vi "2ComboKeyDetect (SubVI).vi"(9 "negKey":T1(ring), 10 "posKey":T1(ring), 11 "keys pressed":T2(array[ring])) -> (3 "speedout":dbl(slide) scale=-100.0..100.0)   [LabVIEW 2018]
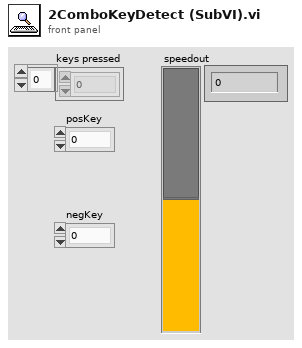
[diagram p1: front panel]
types:
  T1 = enum16{"0", "1", "2", "3", "4", "5", "6", "7", "8", "9", "A", "B", "C", "D", "E", "F", "G", "H", "I", "J", "K", "L", "M", "N", "O", "P", "Q", "R", "S", "T", "U", "V", "W", "X", "Y", "Z", "F1", "F2", "F3", "F4", "F5", "F6", "F7", "F8", "F9", "F10", "F11", "F12", "F13", "F14", "F15", "ADD", "BACK", "BACKSLASH", "CAPITAL", "COMMA", "DECIMAL", "DELETE", "DIVIDE", "DOWN", "END", "EQUALS", "ESCAPE", "GRAVE (`)", "HOME", "INSERT", "LBRACKET", "LCONTROL", "LEFT", "L ALT", "LSHIFT", "LWIN", "MINUS", "MULTIPLY", "NEXT", "NUMLOCK", "NUMPAD_0", "NUMPAD_1", "NUMPAD_2", "NUMPAD_3", "NUMPAD_4", "NUMPAD_5", "NUMPAD_6", "NUMPAD_7", "NUMPAD_8", "NUMPAD_9", "PAUSE", "PERIOD", "PRIOR (PG UP)", "RBRACKET", "RCONTROL", "RETURN", "RIGHT", "R ALT", "RSHIFT", "RWIN", "SCROLL", "SEMICOLON", "SLASH", "SPACE", "SUBTRACT", "TAB", "UP", "ENTER (num pad)", "' (quote)"}
  T2 = enum16{"0", "1", "2", "3", "4", "5", "6", "7", "8", "9", "A", "B", "C", "D", "E", "F", "G", "H", "I", "J", "K", "L", "M", "N", "O", "P", "Q", "R", "S", "T", "U", "V", "W", "X", "Y", "Z", "F1", "F2", "F3", "F4", "F5", "F6", "F7", "F8", "F9", "F10", "F11", "F12", "F13", "F14", "F15", "ADD", "BACK", "BACKSLASH", "CAPITAL", "COMMA", "DECIMAL", "DELETE", "DIVIDE", "DOWN", "END", "EQUALS", "ESCAPE", "GRAVE (`)", "HOME", "INSERT", "LBRACKET", "LCONTROL", "LEFT", "L ALT", "LSHIFT", "LWIN", "MINUS", "MULTIPLY", "NEXT", "NUMLOCK", "NUMPAD_0", "NUMPAD_1", "NUMPAD_2", "NUMPAD_3", "NUMPAD_4", "NUMPAD_5", "NUMPAD_6", "NUMPAD_7", "NUMPAD_8", "NUMPAD_9", "PAUSE", "PERIOD", "PRIOR (PG UP)", "RBRACKET", "RCONTROL", "RETURN", "RIGHT", "R ALT", "RSHIFT", "RWIN", "SCROLL", "SEMICOLON", "SLASH", "SPACE", "SUBTRACT", "TAB", "UP", "ENTER (num pad)", "' (quote)"}[]
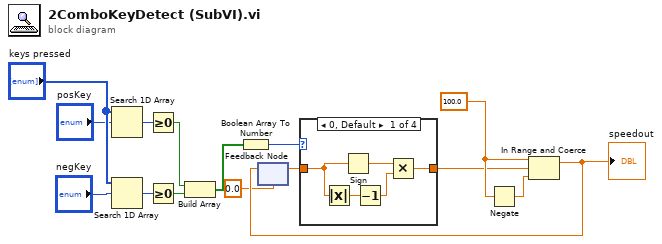
[diagram p0: block diagram]
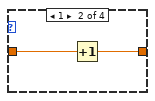
[diagram p2: hidden frame]
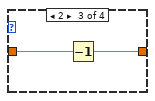
[diagram p3: hidden frame]
diagram:
  w14 = 100.0 ("upper limit")
  n1 = Search 1D Array(1D array="keys pressed", element="posKey") -> (index of element=w2:i32)  [unwired: 1 in]
  n2 = Search 1D Array(1D array="keys pressed", element="negKey") -> (index of element=w3:i32)  [unwired: 1 in]
  n3 = Greater Or Equal To 0?(x=w2) -> (x >= 0?=w6:bool)
  n4 = Greater Or Equal To 0?(x=w3) -> (x >= 0?=w7:bool)
  n5 = Build Array(w6, w7) -> (w8:bool[])
  n6 = Boolean Array To Number(Boolean array=w8) -> (number=w9:u32)
  n7 = feedback #1(0.0) -> (w11:dbl)
  n8 = case shown="0, Default" w9 {
    tunnel: [w17 w21 w23 w25] -> w13
    tunnel: w11 -> [w16 w22 w24 w25]
    frame 0, Default {
      n9 = Absolute Value(x=w16) -> (abs(x)=w20:dbl)
      n10 = Sign(1:w16) -> (0:w18:dbl)
      n11 = Decrement(x=w20) -> (x-1=w19:dbl)
      n12 = Multiply(x=w18, y=w19) -> (x*y=w17:dbl)
    }
    frame 1 {
      n13 = Increment(x=w22) -> (x+1=w21:dbl)
    }
    frame 2 {
      n14 = Decrement(x=w24) -> (x-1=w23:dbl)
    }
    frame 3 {
    }
  }
  n15 = Negate(x=w14) -> (-x=w15:dbl)
  n16 = In Range and Coerce(upper limit=w14, x=w13, lower limit=w15) -> (coerced(x)=w12:dbl)  [unwired: 1 out]
  "speedout" <- w12
  n17 = feedback-in #1(w12) -> ()
